vi "Construct Connection Reader.vi"(5 "Log Alias":string, 7 "Log Instance":refnum<class "LoggerReference.lvclass">, 9 "ProtectedConnection":refnum<class "ProtectedConnectionReader.lvclass">, 10 "ReadStrategy":refnum<class "IReadStrategy.lvclass">, 11 "Message Return Policy":refnum<class "IMessageReturnPolicy.lvclass">) -> (3 "ConnectionReader out":refnum<class "ConnectionReader.lvclass">)   [LabVIEW 2020, in "ConnectionReader.lvlib" / "ConnectionReader.lvclass"]
uses:
  <vilib>/gpm_packages/@cs/Network-interface/Source/ConnectionReader/ConnectionReader/ConnectionReader.lvclass
  C:/Program Files/National Instruments/LabVIEW 2020/vi.lib/gpm_packages/@cs/Network-interface/Source/Logged Actor/LoggedActor.lvclass
  <vilib>/gpm_packages/@cs/Network-interface/Source/ProtectedConnectionReader/ProtectedConnectionReader.lvclass
  <vilib>/gpm_packages/@cs/Network-interface/Source/MessagingInterfaces/IReadStrategy/IReadStrategy.lvclass
  <vilib>/gpm_packages/@cs/Network-interface/Source/MessagingInterfaces/IMessageReturnPolicy/IMessageReturnPolicy.lvclass
  <vilib>/gpm_packages/@cs/event-logger/Source/Composed Log/LoggerReference/LoggerReference.lvclass
  <vilib>/gpm_packages/@cs/Network-interface/Source/ConnectionReader/ConnectionReader/ConnectionReader.lvclass/ConnectionReader.ctl
  <vilib>/gpm_packages/@cs/Network-interface/Source/Logged Actor/LoggedActor.lvclass/LoggedActor.ctl
  <vilib>/gpm_packages/@cs/Network-interface/Source/Logged Actor/LoggedActor.lvclass
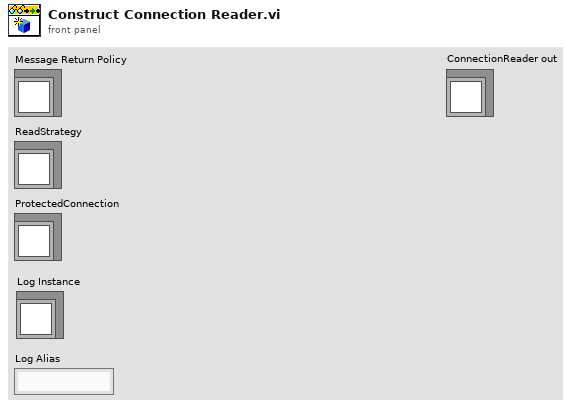
[diagram p1: front panel]
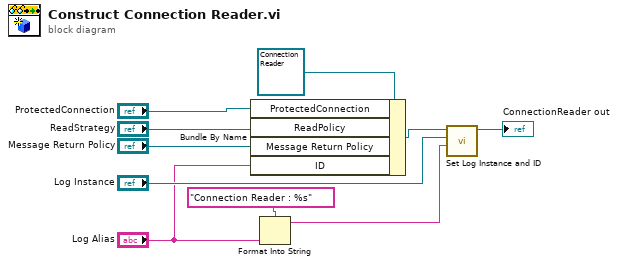
[diagram p0: block diagram]
diagram:
  n1 = Bundle By Name(cluster=refnum<class "ConnectionReader.lvclass"> refnum ("ConnectionReader in"), "ProtectedConnection"="ProtectedConnection", "ReadPolicy"="ReadStrategy", "Message Return Policy"="Message Return Policy", "ID"="Log Alias") -> (w6:refnum<class "ConnectionReader.lvclass">)
  n2 = Format Into String(format string="Connection Reader : %s", "Log Alias") -> (resulting string=w3:string)  [unwired: 2 in, 1 out]
  n3 = call <vilib>:"Set Log Instance and ID.vi"("Log Alias"=w3, "Log Instance"="Log Instance", "LoggedActor in"=w6) -> ("LoggedActor out"=→"ConnectionReader out":refnum<class "ConnectionReader.lvclass">)  [unwired: 8 in]
